vi "7.7-Reliable UDP Server Template.vi"() -> ()   [LabVIEW 2010]
uses:
  3.7 LabVIEW Errors.ctl
  3.0-Global.vi
panel:
  out "Probably a hello string":string
  in  "error in":errorcluster={"status"=TRUE, "code"=0, "source"=""}
  out "error out":errorcluster
  in  "stop":bool
  in  "My Global Variable":cluster{i32, bool}
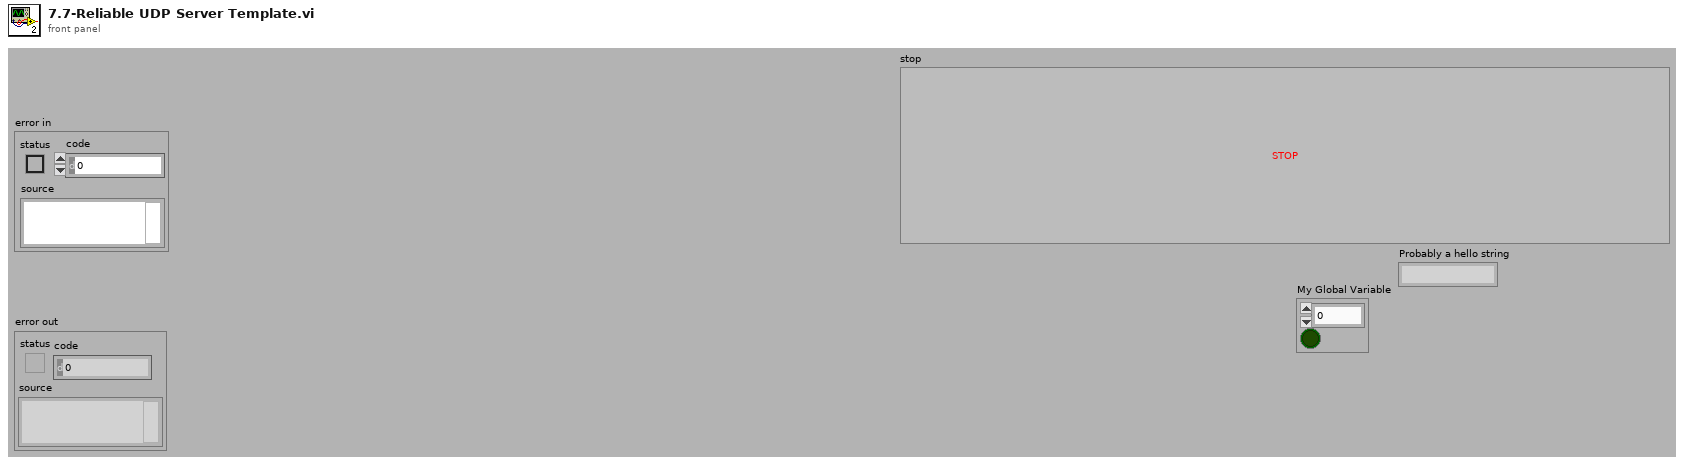
[diagram p1: front panel]
types:
  T1 = typedef "3.7 LabVIEW Errors.ctl" = i32
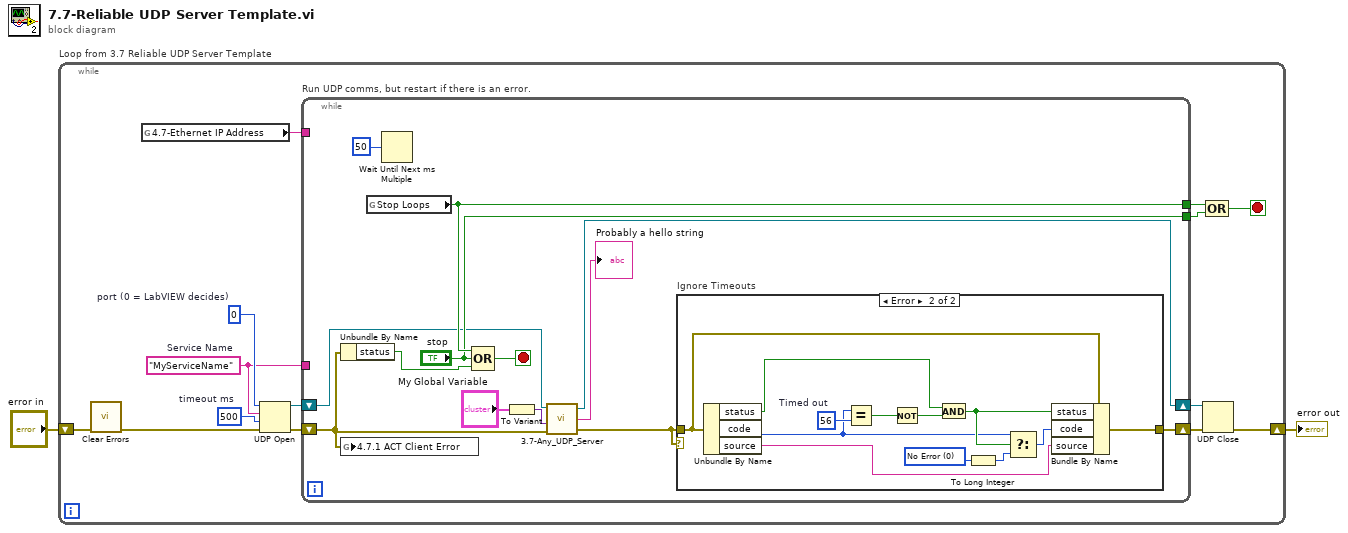
[diagram p0: block diagram]
diagram:
  n1 = while "Loop from 3.7 Reliable UDP Server Template" {
    shift-right: [w9] -> w1
    shift-left: "error in" -> [w5]
    stop <- w14 stop-if-true
    w6 = 500  # timeout ms
    w8 = u16 0  # port (0 = LabVIEW decides)
    w7 = "MyServiceName"  # Service Name
    n2 = call <vilib>:"Clear Errors.vi"("error in (no error)"=w5) -> ("error out"=w4:errorcluster)  [unwired: 6 in]
    n3 = global read "3.0-Global.vi" "4.7-Ethernet IP Address"() -> (w3:string)
    n4 = UDP Open(8:w4, 9:w6, 10:w7, 11:w8) -> (port=w13:refnum<k16>, 0:w11:errorcluster)  [unwired: 1 in, 1 out]
    n5 = while "Run UDP comms, but restart if there is an error." {
      tunnel: w7 -> [_]
      tunnel: w3 -> [_]
      tunnel: [w27] -> w16
      tunnel: ["stop"] -> w15
      shift-right: [w19] -> w12
      shift-left: w13 -> [w20]
      shift-right: [w24] -> w10
      shift-left: w11 -> [w22]
      stop <- w29 stop-if-true
      n6 = Unbundle By Name(w22) -> ("status"=w25:bool)
      n7 = global write "3.0-Global.vi" "4.7.1 ACT Client Error"(w22) -> ()
      n8 = global read "3.0-Global.vi" "Stop Loops"() -> (w27:bool)
      n9 = Wait Until Next ms Multiple(millisecond multiple=u32 50) -> ()  [unwired: 1 out]
      n10 = Compound Arithmetic op=OR(w27, "stop", w25) -> (w29:bool)
      n11 = To Variant(anything="My Global Variable") -> (Variant=w18:variant)
      n12 = call "3.7-Any_UDP_Server.vi"("error In"=w22, "Data in"=w18, "Connection ID"=w20) -> ("warning out"=w21:errorcluster, "data out"=→"Probably a hello string":string, "Connection ID out"=w19:refnum<k16>)  [unwired: 1 in]
      n13 = case "Ignore Timeouts" shown="Error" w21 {
        tunnel: w21 -> [w30 w42]
        tunnel: [w30 w41] -> w24
        frame No Error {
        }
        frame Error {
          w32 = T1 0 items=["No Error", "Argument Error", "Memory Full", "Out of Zone", "End of File", "File Already Open", "Generic File IO Error", "File Not Found", "File Permission Error", "Disk Full", "Duplicate Path", "Too Many Files Open", "Not Enabled", "Resource File Not Found", "Cannot Add Resource", "Resource Not Found", "Image Not Found", "Image Memory Error", "Pen Does Not Exist", "Config Bad Type", "Config Token Not Found", "Config Parse Error", "Config Memory Error", "Bad External Code Format", "Bad External Code Offset", "External Code Not Present", "Null Window", "Destroy Window Mixup", "Null Menu", "Print Aborted", "Bad Print Record", "Print Driver Error", "Windows Error During Print", "Memory Error During Print", "Print Dialog Error", "Generic Print Error", "Invalid Device Refnum", "Device Not Found", "Device Parameter Error", "Device Unit Error", "Can't Open Device", "Device Call Aborted", "Generic Error", "Cancelled By User", "Object ID Too Low", "Object ID Too High", "Object Not In Heap", "Unknown Heap", "Bad DefProc ID", "DefProc Not In Table", "Message Out Of Range", "Null Method", "Unknown Message", "Manager Call Not Supported", "Bad address", "Connection In progress", "Connection timed out", "Connection is already in progress", "Network attribute not supported", "Network error", "Address in use", "System out of memory", "Connection aborted", "Connection refused", "Connection is not connected", "Connection is already connected", "Connection closed", "Initialize error (interapplication manager)", "Bad occurrence", "Wait on unbound occurrence handler", "Occurrence queue overflow", "Bad path", "Semaphore not signaled", "Unrecognized type (interapplication manager)"] ("1st Error to Convert")
          w40 = 56  # Timed out
          n14 = Unbundle By Name(w42) -> ("status"=w37:bool, "code"=w35:i32, "source"=w33:string)
          n15 = Equal?(x=w35, y=w40) -> (x = y?=w39:bool)
          n16 = Not(x=w39) -> (.not. x?=w38:bool)
          n17 = And(x=w37, y=w38) -> (x .and. y?=w36:bool)
          n18 = To Long Integer(number=w32) -> (32bit integer=w31:T1)
          n19 = Select(t=w35, s=w36, f=w31) -> (s? t:f=w34:T1)
          n20 = Bundle By Name(cluster=w42, "status"=w36, "code"=w34, "source"=w33) -> (w41:errorcluster)
        }
      }
    }
    n21 = UDP Close(connection ID=w12, 8:w10) -> (error out=w9:errorcluster)  [unwired: 1 out]
    n22 = Compound Arithmetic op=OR(w16, w15) -> (w14:bool)
  }
  "error out" <- w1
